vi "Read Available Disk Space.vi"(8 "error in (no error)":errorcluster, 11 "VISA resource name":refnum<visa-resource-name>) -> (0 "error out":errorcluster, 2 "Available Space":i32, 3 "VISA resource name out":refnum<visa-resource-name>)   [LabVIEW 2010, in "Temptronic TP04300.lvlib"]
doc: "This VI reads the remaining disk space available for datalogging in bytes.\n\nNote: The maximum space value returned is limited to 2147483647 bytes (2 Gbytes)"
uses:
  Temptronic TP04300.lvlib
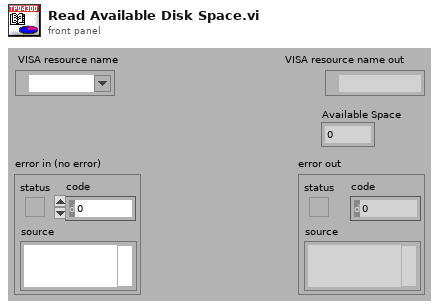
[diagram p1: front panel]
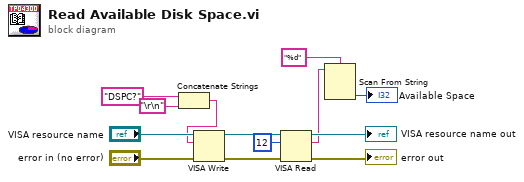
[diagram p0: block diagram]
diagram:
  n1 = Concatenate Strings("DSPC?" ("multi-line string"), "\r\n") -> (w3:string)
  n2 = VISA Write(VISA resource name="VISA resource name", write buffer=w3, error in (no error)="error in (no error)") -> (VISA resource name out=w11:refnum<visa-resource-name>, error out=w9:errorcluster)  [unwired: 1 out]
  n3 = VISA Read(VISA resource name=w11, byte count=u32 12, error in (no error)=w9) -> (VISA resource name out=→"VISA resource name out":refnum<visa-resource-name>, read buffer=w4:string, error out=→"error out":errorcluster)  [unwired: 1 out]
  n4 = Scan From String(format string="%d", input string=w4) -> (output 1=→"Available Space":i32)  [unwired: 3 in, 3 out]
